vi "N6701A_SetCurrent.vi"(6 "Behavior (0: Regulatory Limit)":i32(ring) items=["Regulatory Limit", "Trip Limit"], 8 "error in (no error)":errorcluster, 9 "Limit (0.0 amps)":dbl format="%^.3e", 10 "Channel Name (1)":string="1", 11 "VISA resource name":refnum<visa-resource-name>) -> (0 "error out":errorcluster)   [LabVIEW 2015]
uses:
  <instrlib>/Agilent N6700 Series/Agilent N6700 Series.lvlib
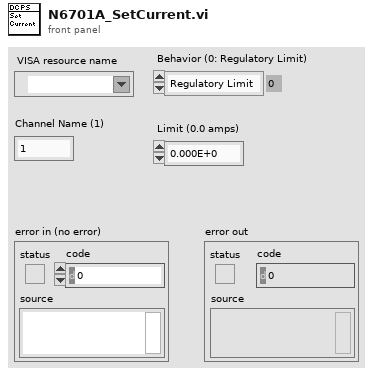
[diagram p1: front panel]
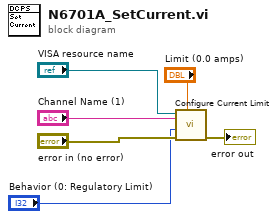
[diagram p0: block diagram]
diagram:
  n1 = call <instrlib>:"Configure Current Limit.vi"("Limit (0.0 amps)"="Limit (0.0 amps)", "error in (no error)"="error in (no error)", "Behavior (0: Regulatory Limit)"="Behavior (0: Regulatory Limit)", "Channel Name (1)"="Channel Name (1)", "VISA resource name"="VISA resource name") -> ("error out"=→"error out":errorcluster)  [unwired: 5 in, 1 out]
